vi "Find Aliases and Routes.vi"(8 "error in (no error)":errorcluster, 11 "RaF CD Ref in":T1 format="%.0x") -> (0 "error out":errorcluster, 1 "Aliases Section Ref":T1 format="%.0x", 2 "Routes Section Ref":T1 format="%.0x", 3 "RaF CD Ref out":T1 format="%.0x")   [LabVIEW 2017, in "Switch Scripting.lvlib"]
uses:
  Switch Scripting.lvlib
  <vilib>/NI Veristand/Custom Device API/Custom Device Item Ref.ctl
  NationalInstruments.VeriStand.SystemDefinitionAPI
  Shared/Constants.vi
  Shared/Switch Shared.lvlib
  <vilib>/NI VeriStand/Custom Device API/Custom Device API.lvlib
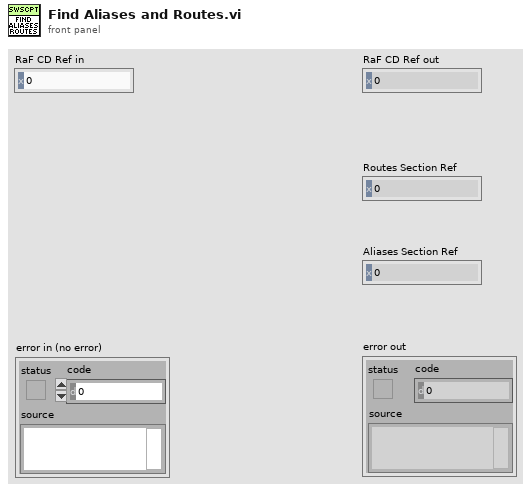
[diagram p1: front panel]
types:
  T1 = typedef "Custom Device API.lvlib/Custom Device Item Ref.ctl" = u64
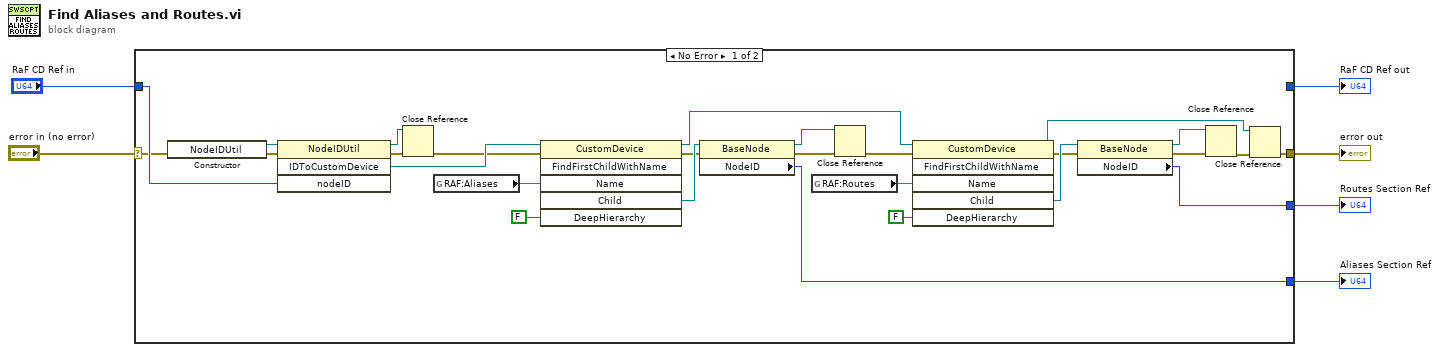
[diagram p0: block diagram]
diagram:
  n1 = case shown="No Error" "error in (no error)" {
    selector: "error in (no error)" -> [w17 w35]
    tunnel: "RaF CD Ref in" -> [w19 w34]
    tunnel: [_ w34] -> w5
    tunnel: [w27 _] -> w4
    tunnel: [w8 w35] -> w3
    tunnel: [w24 _] -> w2
    frame No Error {
      n2 = constructor class="NodeIDUtil"(error in=w17) -> (reference out=w20:refnum<k24>, error out=w21:errorcluster)  [unwired: 2 in, 1 out]
      n3 = invoke class="NodeIDUtil" method="IDToCustomDevice"(reference=w20, error in=w21, "nodeID"=w19) -> (reference out=w15:refnum<k24>, error out=w16:errorcluster, "IDToCustomDevice"=w18:refnum<k24>)  [unwired: 1 in, 1 out]
      n4 = Close Reference(reference=w15, error in (no error)=w16) -> (error out=w14:errorcluster)
      n5 = global read "Constants.vi" "RAF:Aliases"() -> (w33:string)
      n6 = invoke class="CustomDevice" method="FindFirstChildWithName"(reference=w18, error in=w14, "Name"=w33, "DeepHierarchy"=FALSE) -> (reference out=w10:refnum<k24>, error out=w30:errorcluster, "Child"=w32:refnum<k24>)  [unwired: 2 in, 3 out]
      n7 = property class="BaseNode"(reference=w32, error in=w30) -> (reference out=w12:refnum<k24>, error out=w13:errorcluster, "NodeID"=w24:u64)
      n8 = global read "Constants.vi" "RAF:Routes"() -> (w29:string)
      n9 = Close Reference(reference=w12, error in (no error)=w13) -> (error out=w11:errorcluster)
      n10 = invoke class="CustomDevice" method="FindFirstChildWithName"(reference=w10, error in=w11, "Name"=w29, "DeepHierarchy"=FALSE) -> (reference out=w7:refnum<k24>, error out=w28:errorcluster, "Child"=w31:refnum<k24>)  [unwired: 2 in, 3 out]
      n11 = property class="BaseNode"(reference=w31, error in=w28) -> (reference out=w22:refnum<k24>, error out=w23:errorcluster, "NodeID"=w27:u64)
      n12 = Close Reference(reference=w22, error in (no error)=w23) -> (error out=w9:errorcluster)
      n13 = Close Reference(reference=w7, error in (no error)=w9) -> (error out=w8:errorcluster)
    }
    frame Error {
    }
  }
  "RaF CD Ref out" <- w5
  "Aliases Section Ref" <- w2
  "Routes Section Ref" <- w4
  "error out" <- w3
